vi "OxITC503 _Query_ Read Command.vi"(3 "error in":errorcluster, 4 "Read Item":T1(ring), 5 "VISA session":refnum<visa-resource-name>) -> (0 "error out (no error)":errorcluster, 1 "Output of Read":dbl format="%.2f", 2 "VISA session":refnum<visa-resource-name>)   [LabVIEW 2014]
doc: "Sends a READ command (Rn) to the ITC 503, that allows the application to query any of the variables listed in the \"Read Item\" menu."
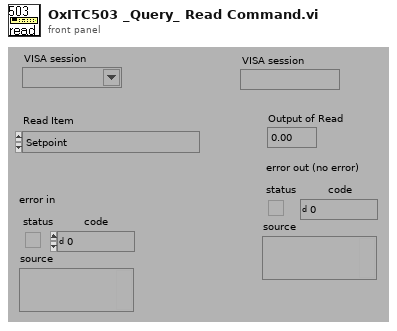
[diagram p1: front panel]
types:
  T1 = enum16{"Setpoint", "Sensor 1", "Sensor 2", "Sensor 3", "Temperature Error", "Heater Output (%)", "Heater Output (V)", "Gas Flow Output", "P Term", "I term", "D term", "Channel 1 Frequency/4", "Channel 2 Frequency/4", "Channel 3 Frequency/4"}
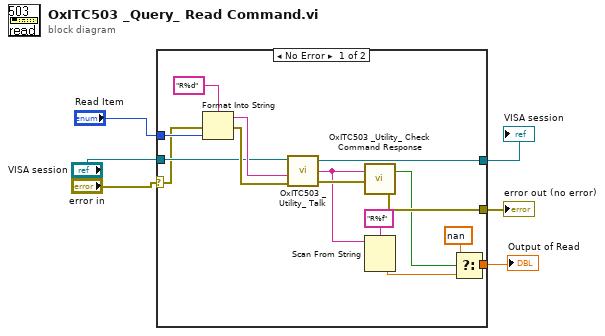
[diagram p0: block diagram]
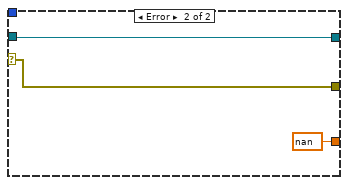
[diagram p2: hidden frame]
diagram:
  n1 = case shown="No Error" "error in" {
    selector: "error in" -> [w7 w23]
    tunnel: [w21 w23] -> w6
    tunnel: [w16 w22] -> w5
    tunnel: "VISA session" -> [w15 w22]
    tunnel: "Read Item" -> [w14 _]
    tunnel: [w9 nan ("t")] -> w2
    frame No Error {
      n2 = Format Into String(format string="R%d" ("Format String"), error in=w7, w14) -> (resulting string=w18:string, error out=w19:errorcluster)  [unwired: 1 in]
      n3 = call "OxITC503 _Utility_ Talk.vi"("VISA session"=w15, "Command"=w18, "error in (no error)"=w19) -> ("VISA session"=w16:refnum<visa-resource-name>, "read buffer"=w13:string, "error out (no error)"=w20:errorcluster)  [unwired: 2 in]
      n4 = call "OxITC503 _Utility_ Check Command Response.vi"("error in"=w20, "read buffer"=w13) -> ("error out (no error)"=w21:errorcluster, "Error occurred?"=w11:bool)
      n5 = Scan From String(format string="R%f" ("Format String"), input string=w13) -> (output 1=w10:dbl)  [unwired: 3 in, 3 out]
      n6 = Select(t=nan, s=w11, f=w10) -> (s? t:f=w9:dbl)
    }
    frame Error {
    }
  }
  "error out (no error)" <- w6
  "VISA session" <- w5
  "Output of Read" <- w2
